vi "Absolute Encoder Read.vi"(8 "Error":errorcluster, 11 "Cluster":T1) -> (0 "Error Out":errorcluster, 1 "Total Encoder Counts Out":i32, 2 "Single Encoder Counts Out":i32, 3 "Cluster Out":T1, 4 "Count Out":i32, 5 "Total Revolution Out":dbl, 7 "Single Revolution Out":dbl)   [LabVIEW 2023]
uses:
  Cluster_Absolute Encoder Ref.ctl
  <vilib>/Rock Robotics/SystemInterfaces/DutyCycle/FPGA_DutyCycleDevRef.ctl
  <vilib>/Rock Robotics/SystemInterfaces/DutyCycle/FPGA_DutyCycleIndex.ctl
  <vilib>/Rock Robotics/WPI/Counter/WPI_CounterDevRef.ctl
  <vilib>/Rock Robotics/SystemInterfaces/Counter/FPGA_CounterCtrSystemIndex.ctl
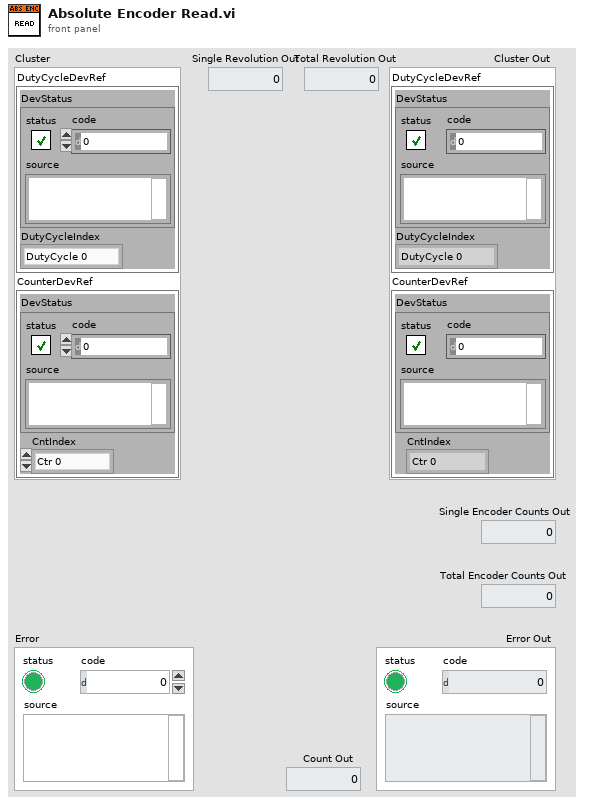
[diagram p1: front panel]
types:
  T1 = typedef "Cluster_Absolute Encoder Ref.ctl" = cluster{"DutyCycleDevRef":T2, "CounterDevRef":T4}
  T2 = typedef "FPGA_DutyCycleDevRef.ctl" = cluster{"DevStatus":errorcluster, "DutyCycleIndex":T3}
  T3 = typedef "FPGA_DutyCycleIndex.ctl" = enum8{"DutyCycle 0", "DutyCycle 1", "DutyCycle 2", "DutyCycle 3", "DutyCycle 4", "DutyCycle 5", "DutyCycle 6", "DutyCycle 7", "Invalid"}
  T4 = typedef "WPI_CounterDevRef.ctl" = cluster{"DevStatus":errorcluster, "CntIndex":T5}
  T5 = typedef "FPGA_CounterCtrSystemIndex.ctl" = enum8{"Ctr 0", "Ctr 1", "Ctr 2", "Ctr 3", "Ctr 4", "Ctr 5", "Ctr 6", "Ctr 7", "Invalid"}
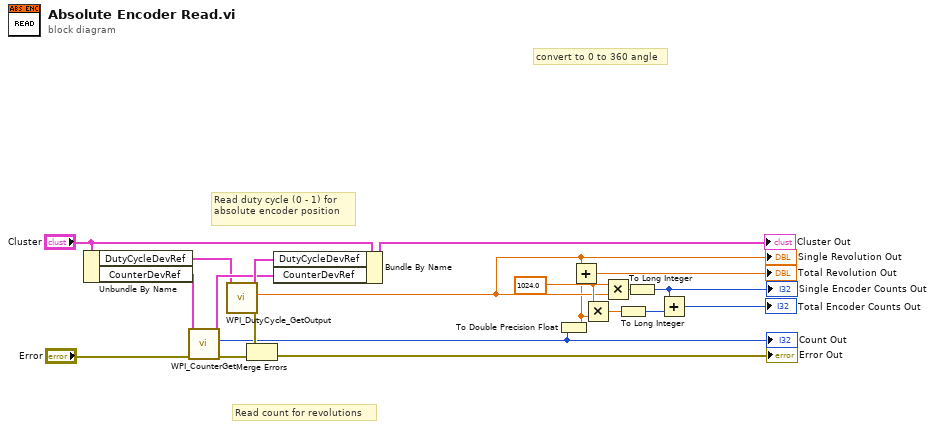
[diagram p0: block diagram]
diagram:
  w9 = 1024.0 ("x")
  # "Read count for revolutions"
  # "Read duty cycle (0 - 1) for absolute encoder position"
  # "convert to 0 to 360 angle"
  n1 = Unbundle By Name("Cluster") -> ("DutyCycleDevRef"=w15:T2, "CounterDevRef"=w16:T4)
  n2 = call <vilib>:"WPI_CounterGet.vi"("error in (no error)"="Error", "CounterDevRef in"=w16) -> ("error out"=w11:errorcluster, "Value"=w1:i32, "CounterDevRef out"=w17:T4)  [unwired: 4 in, 3 out]
  "Count Out" <- w1
  n3 = call <vilib>:"WPI_DutyCycle_GetOutput.vi"("DutyCycleDevRef"=w15) -> ("error out"=w12:errorcluster, "Output"=w5:dbl, "DutyCycleDevRef Out"=w18:T2)  [unwired: 8 in]
  "Single Revolution Out" <- w5
  n4 = Merge Errors(w12, w11) -> (→"Error Out":errorcluster)
  n5 = Bundle By Name(cluster="Cluster", "DutyCycleDevRef"=w18, "CounterDevRef"=w17) -> (→"Cluster Out":T1)
  n6 = To Double Precision Float(number=w1) -> (double precision float=w2:dbl)
  n7 = Add(x=w5, y=w2) -> (x+y=→"Total Revolution Out":dbl)
  n8 = Multiply(x=w9, y=w2) -> (x*y=w8:dbl)
  n9 = Multiply(x=w9, y=w5) -> (x*y=w7:dbl)
  n10 = To Long Integer(number=w8) -> (32bit integer=w3:i32)
  n11 = To Long Integer(number=w7) -> (32bit integer=w4:i32)
  "Single Encoder Counts Out" <- w4
  n12 = Add(x=w4, y=w3) -> (x+y=→"Total Encoder Counts Out":i32)
